vi "Find index.vi"(10 "Frequency (GHz)":dbl, 11 "Power readings":cluster{"Frequency":dbl, "Power":dbl}[](array[cluster])) -> (3 "Index of matching or greater point":i32)   [LabVIEW 2018, in "Power control.lvclass"]
uses:
  Power control.lvclass
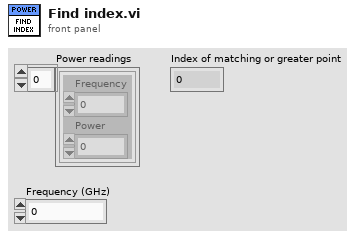
[diagram p1: front panel]
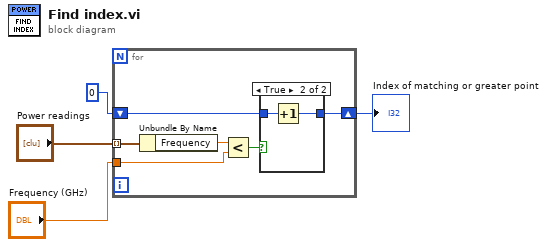
[diagram p0: block diagram]
diagram:
  n1 = for {
    shift-right: [w5] -> w3
    shift-left: 0 -> [w6]
    tunnel: "Power readings" -> [w10] mode=indexing
    tunnel: "Frequency (GHz)" -> [w8]
    n2 = Unbundle By Name(w10) -> ("Frequency"=w9:dbl)
    n3 = Less?(x=w9, y=w8) -> (x < y?=w7:bool)
    n4 = case shown="True" w7 {
      tunnel: w6 -> [w11 w13]
      tunnel: [w11 w12] -> w5
      frame False {
      }
      frame True {
        n5 = Increment(x=w13) -> (x+1=w12:i32)
      }
    }
  }
  "Index of matching or greater point" <- w3
